vi "CreateJoystickEvent.vi"(5 "error in":errorcluster) -> (16 "Joystick event":T1, 19 "error out":errorcluster)   [LabVIEW 2018]
uses:
  Joystick event.ctl
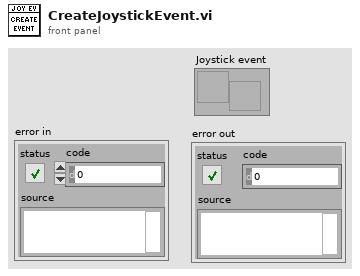
[diagram p1: front panel]
types:
  T1 = typedef "Joystick event.ctl" = refnum<user-event>
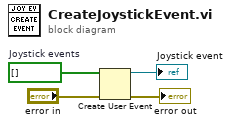
[diagram p0: block diagram]
diagram:
  w4 = bool[] []  # Joystick events
  n1 = Create User Event(user event datatype=w4, error in="error in") -> (user event=→"Joystick event":refnum<user-event>, error out=→"error out":errorcluster)
